vi "startTest.vi"(8 "error in (no error)":errorcluster, 10 "model":refnum<class "Model.lvclass">, 11 "StoppedState in":refnum<class "StoppedState.lvclass">) -> (0 "error out":errorcluster, 2 "model 2":refnum<class "Model.lvclass">, 3 "StoppedState out":refnum<class "StoppedState.lvclass">)   [LabVIEW 2013, in "StoppedState.lvclass"]
uses:
  StoppedState.lvclass
  Model/Model/Model.lvclass
  Typedefs/StateSelector.ctl
  EnabledState/EnabledState.lvclass
  Typedefs/AITDTTypedefs.lvlib
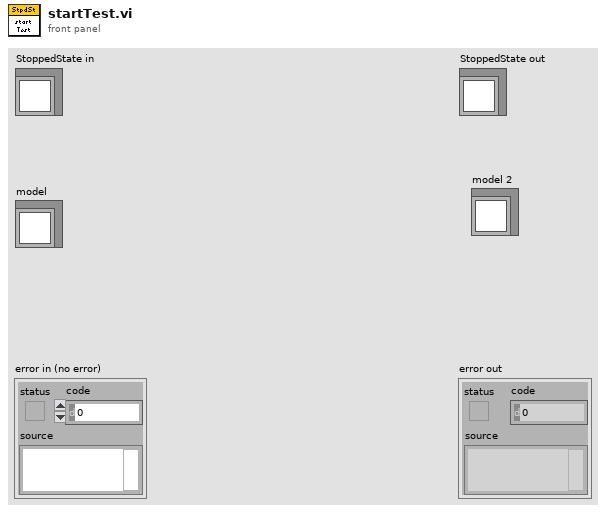
[diagram p1: front panel]
types:
  T1 = typedef "AITDTTypedefs.lvlib/StateSelector.ctl" = enum16{"AwaitingSetpointAcknowledgmentState", "EndingCycleState", "FaultState", "OffState", "PausingState", "RequestingNewSetpointState", "SamplingState", "SettlingState", "SoakingState", "StabilizingState", "StandbyState", "StoppedState", "TransitioningTemperatureState"}
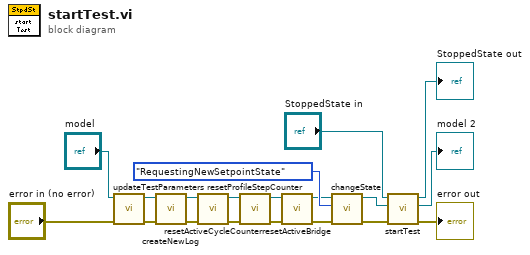
[diagram p0: block diagram]
diagram:
  n1 = call "updateTestParameters.vi"("error in (no error)"="error in (no error)", "Model in"="model") -> ("error out"=w9:errorcluster, "Model out"=w11:refnum<class "Model.lvclass">)  [unwired: 8 in]
  n2 = call "createNewLog.vi"("error in (no error)"=w9, "Model in"=w11) -> ("error out"=w6:errorcluster, "Model out"=w8:refnum<class "Model.lvclass">)  [unwired: 8 in]
  n3 = call "resetActiveCycleCounter.vi"("error in (no error)"=w6, "Model in"=w8) -> ("error out"=w5:errorcluster, "Model out"=w7:refnum<class "Model.lvclass">)  [unwired: 8 in]
  n4 = call "resetProfileStepCounter.vi"("error in (no error)"=w5, "Model in"=w7) -> ("error out"=w3:errorcluster, "Model out"=w4:refnum<class "Model.lvclass">)  [unwired: 8 in]
  n5 = call "resetActiveBridge.vi"("error in (no error)"=w3, "Model in"=w4) -> ("error out"=w1:errorcluster, "Model out"=w2:refnum<class "Model.lvclass">)  [unwired: 8 in]
  n6 = call "changeState.vi"("error in (no error)"=w1, "State:"=StateSelector."RequestingNewSetpointState", "Model in"=w2) -> ("error out"=w13:errorcluster, "Model out"=w14:refnum<class "Model.lvclass">)  [unwired: 7 in]
  n7 = call-parent "startTest.vi"("error in (no error)"=w13, "model"=w14, "State in"="StoppedState in") -> ("error out"=→"error out":errorcluster, "model 2"=→"model 2":refnum<class "Model.lvclass">, "State out"=→"StoppedState out":refnum<class "StoppedState.lvclass">)  [unwired: 6 in]
